vi "MT_connect_real_1.vi"() -> ()   [LabVIEW 2017]
uses:
  <vilib>/regexp/Match Regular Expression.xnode
  <vilib>/addons/internet/NI_InternetTK_Core_VIs.lvlib
panel:
  out "concatenated string":string
  out "content 5":string
  out "content 4":string
  out "empty? 2":bool
  in  "Machine 2":string="NMV8000"
  in  "MT Connect Agent 2":string="http://amrcmtconnect.shef.ac.uk:5000/"
  out "after match 2":string
  out "content1 2":string
  out "concatenated string 2":string
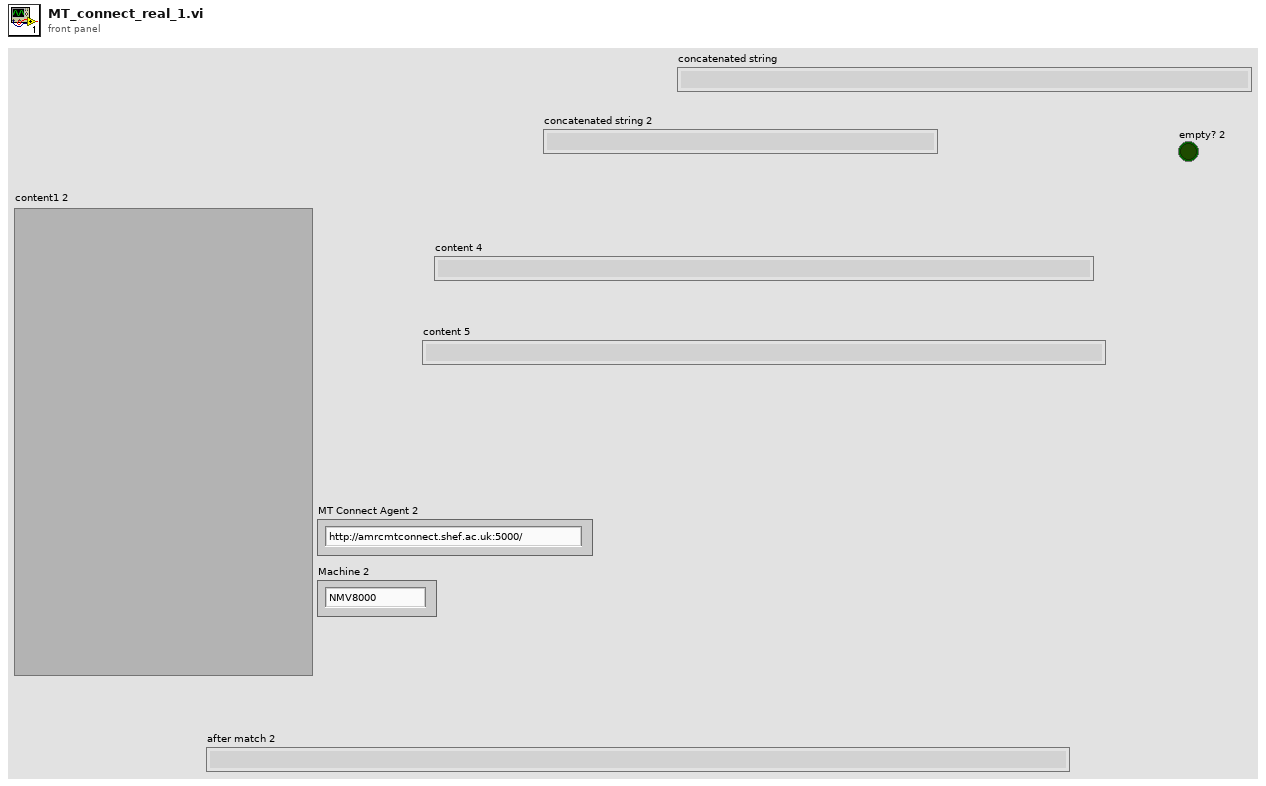
[diagram p1: front panel]
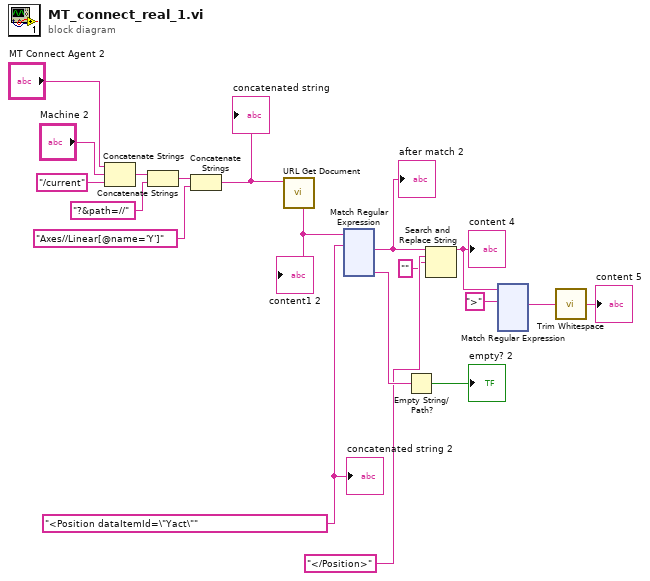
[diagram p0: block diagram]
diagram:
  w1 = "<Position dataItemId=\"Yact\"" ("regular expression")
  n1 = Concatenate Strings("MT Connect Agent 2", "Machine 2", "/current" ("string")) -> (w11:string)
  n2 = Concatenate Strings(w11, "?&path=//" ("string")) -> (w12:string)
  n3 = Concatenate Strings(w12, "Axes//Linear[@name='Y']" ("string")) -> (w8:string)
  "concatenated string" <- w8
  n4 = call <vilib>:"URL Get Document.vi"("URL"=w8) -> ("content"=w15:string)  [unwired: 6 in, 4 out]
  "content1 2" <- w15
  n5 = xnode "Match Regular Expression"("input string"=w15, "regular expression"=w1) -> ("after match"=w16:string, "submatch 1"=w13:string)  [unwired: 4 in, 4 out]
  "after match 2" <- w16
  n6 = Empty String/Path?(string/path=w13) -> (empty?=→"empty? 2":bool)
  n7 = Search and Replace String(input string=w16, search string="</Position>" ("string"), replace string="" ("string")) -> (result string=w17:string)  [unwired: 5 in, 3 out]
  "content 4" <- w17
  n8 = xnode "Match Regular Expression"("input string"=w17, "regular expression"=">" ("string")) -> ("after match"=w18:string)  [unwired: 4 in, 5 out]
  n9 = call <vilib>:"Trim Whitespace.vi"("string"=w18) -> ("trimmed string"=→"content 5":string)  [unwired: 1 in]
  "concatenated string 2" <- w1
